vi "Packet Testing.vi"(7 "Send":bool, 8 "error in (no error)":errorcluster) -> (0 "Error Out":errorcluster)   [LabVIEW 2015]
uses:
  Type/TCP Packet Info.ctl
  Type/_RT Command.ctl
panel:
  out "Requested Sequence Number":i32
  out "Response Sequence Number":i32
  out "Response Packet Signature":string
  in  "Command":T1=enum."Get Status"
  in  "Packet Signature":string="RQ"
  in  "Data Message Size":u32
  in  "Data Message":string
  in  "Checksum":u32=18
  out "Error Message":string
  in  "Packet Info In":T2={"Packet Signature"="", "Sequence Number"=0, "Command"=enum."xml Set LC Input Logic", "Data Message Size"=0, "Data Message Size"="", "Data Message"="", "Error Message Size"=0, "Error Message Size"="", "Error Message"="", "Checksum"=0, "Error Message"={"status"=FALSE, "code"=0, "source"=""}, "Command ID"=""}
  out "Data Message":string
  in  "stop":bool
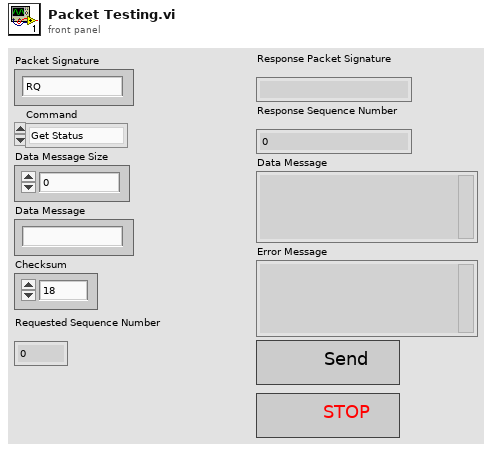
[diagram p1: front panel]
types:
  T1 = typedef "_RT Command.ctl" = enum16{"xml Start Run", "xml Start Actual Run", "xml Stop Run", "xml Runtime Update", "xml Get Status", "xml Get Table", "xml Set Table", "xml Get Configuration", "xml System Status", "xml Set LC Input Logic", "xml Get Data", "xml Get Info", "Start", "StartActualRun", "Stop", "Runtime Update", "Get Data", "Get Info", "Get Status", "Get Param", "Get Config", "Get Table", "Read ADC", "Set Oscillator", "Update Config", "Update Table", "Set All Pol", "Set Pol and DC", "Set Max Mass", "Toggle RP", "Toggle EL", "Set PIC", "Initialize Turbo", "Send Turbo Comm", "Close Turbo", "P1", "P2", "P3", "Send Serial", "Set LC Out", "Get LC In", "Read VAC", "Test Table", "Toggle Power", "Get Startup", "Set Startup", "Get ADC Table", "Set ADC Table", "Get Brief Status", "Get Detail Status", "Auxiliary Update", "Set CC Logics", "Set CC Input Logics", "Ignore Error", "invalid"}
  T2 = typedef "TCP Packet Info.ctl" = cluster{"Packet Signature":string, "Sequence Number":i32, "Command":T1, "Data Message Size":u32, "Data Message Size":string, "Data Message":string, "Error Message Size":u32, "Error Message Size":string, "Error Message":string, "Checksum":u32, "Error Message":errorcluster, "Command ID":string}
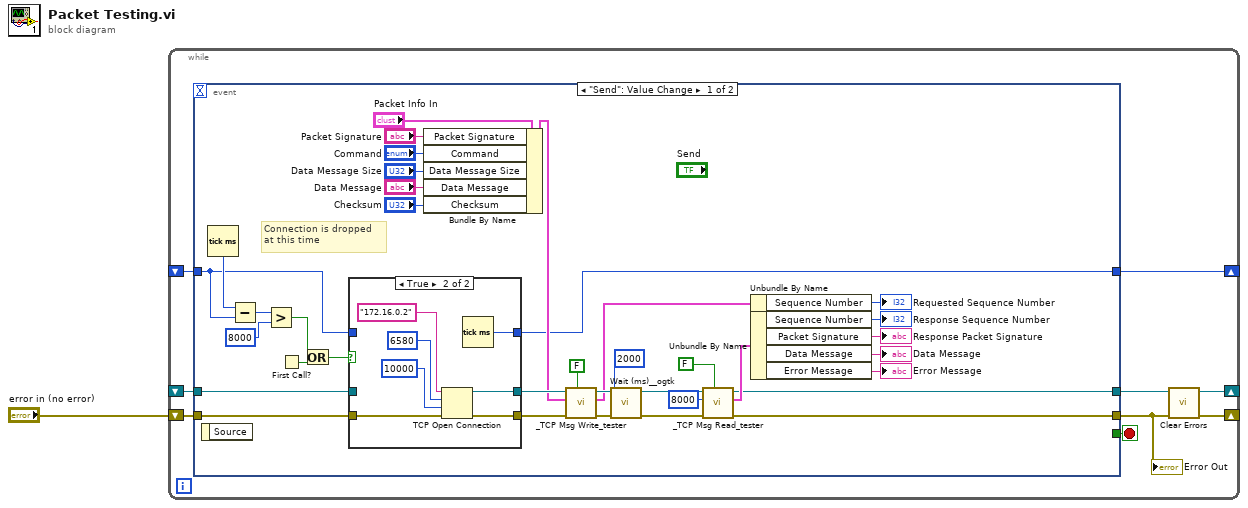
[diagram p0: block diagram]
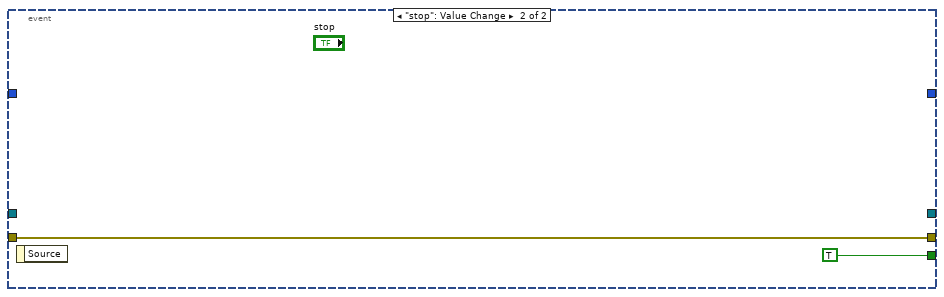
[diagram p3: hidden frame]
diagram:
  n1 = while {
    shift-right: [w8] -> _
    shift-left: "error in (no error)" -> [w9]
    shift-right: [w5] -> _
    shift-left: _ -> [w4]
    shift-right: [w3] -> _
    shift-left: _ -> [w2]
    stop <- w7 stop-if-true
    n2 = event shown="[0] \"Send\": Value Change" {
      selector: _ -> [_ _]
      dyn-events: _ -> [_ _]
      timeout: _ -> [_ _]
      tunnel: w9 -> [w42 w55]
      tunnel: [_ TRUE ("stop")] -> w7
      tunnel: [w35 w55] -> w6
      tunnel: [w19 _] -> w5
      tunnel: w4 -> [w18 _]
      tunnel: [w16 _] -> w3
      tunnel: w2 -> [w10 _]
      event "Send": Value Change {
        # "Connection is dropped\nat this time"
        n3 = event-data() -> ()  [unwired: 1 in, 1 out]
        n4 = Tick Count (ms)() -> (millisecond timer value=w15:u32)
        n5 = Subtract(x=w15, y=w10) -> (x-y=w14:u32)
        n6 = Greater?(x=w14, y=u32 8000) -> (0:w12:bool)
        n7 = First Call?() -> (First Call?: T/F=w17:bool)
        n8 = Or(x=w12, y=w17) -> (x .or. y?=w11:bool)
        n9 = case shown="True" w11 {
          tunnel: w42 -> [w46 w51]
          tunnel: [w46 w50] -> w41
          tunnel: [w47 w49] -> w40
          tunnel: w18 -> [w47 _]
          tunnel: [w45 w48] -> w16
          tunnel: w10 -> [w45 _]
          frame False {
          }
          frame True {
            n10 = TCP Open Connection(address="172.16.0.2", remote port or service name=u16 6580, timeout ms (60000)=10000, error in (no error)=w51) -> (connection ID=w49:refnum<k5>, error out=w50:errorcluster)  [unwired: 1 in]
            n11 = Tick Count (ms)() -> (millisecond timer value=w48:u32)
          }
        }
        n12 = Bundle By Name(cluster="Packet Info In", "Packet Signature"="Packet Signature", "Command"="Command", "Data Message Size"="Data Message Size", "Data Message"="Data Message", "Checksum"="Checksum") -> (w29:T2)
        n13 = call "_TCP Msg Write_tester.vi"("RT"=FALSE, "error in"=w41, "Packet Info In"=w29, "connection ID In"=w40) -> ("error out"=w36:errorcluster, "Packet Info In Out"=w21:T2, "connection ID out"=w37:refnum<k5>)  [unwired: 5 in]
        n14 = call <userlib>:"Wait (ms)__ogtk.vi"("error in (no error)"=w36, "milliseconds to wait"=u32 2000) -> ("error out"=w31:errorcluster)  [unwired: 8 in, 1 out]
        n15 = call "_TCP Msg Read_tester.vi"("RT"=FALSE, "error in"=w31, "timeout ms (10000)"=8000 ("millisecond multiple"), "connection ID"=w37) -> ("error out"=w35:errorcluster, "Packet Info"=w34:T2, "connection ID out"=w19:refnum<k5>)  [unwired: 4 in, 1 out]
        n16 = Unbundle By Name(w21) -> ("Sequence Number"=→"Requested Sequence Number":i32)
        n17 = Unbundle By Name(w34) -> ("Sequence Number"=→"Response Sequence Number":i32, "Packet Signature"=→"Response Packet Signature":string, "Data Message"=→"Data Message":string, "Error Message"=→"Error Message":string)
      }
      event "stop": Value Change {
        n18 = event-data() -> ()  [unwired: 1 in, 1 out]
      }
    }
    "Error Out" <- w6
    n19 = call <vilib>:"Clear Errors.vi"("error in (no error)"=w6) -> ("error out"=w8:errorcluster)  [unwired: 5 in, 1 out]
  }
